vi "Motors Values.vi"() -> ()   [LabVIEW 2012]
panel:
  in  "Feeder":dbl
  in  "Canenet Right+Left":dbl
  in  "Climb Telescopic Right+Left":dbl
  in  "zAvit":dbl
  in  "Second Cannon":dbl
  in  "First Cannon":dbl
  in  "Transfer":dbl
  in  "Flipper":dbl
  in  "Conveyer Belt":dbl
  in  "Roller":dbl
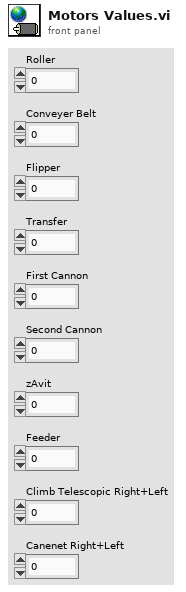
[diagram p1: front panel]
diagram:
